vi "Set Ao.vi"(8 "error in (no error)":errorcluster, 9 "Indx":i32, 10 "Value":dbl, 11 "FPGA_Concrete in":refnum<class "FPGA_Concrete.lvclass">) -> (0 "error out":errorcluster, 3 "FPGA_Concrete out":refnum<class "FPGA_Concrete.lvclass">)   [LabVIEW 2019, in "FPGA_Concrete.lvclass"]
uses:
  FPGA_Concrete.lvclass
  FPGA_Concrete.lvclass/FPGA_Concrete.ctl
  <vilib>/Utility/error.llb/Error Cluster From Error Code.vi
  <vilib>/rvi/errors/niLvFpgaAdjustHostInterfaceError.vi
  <vilib>/ErrorRing/Error Ring.xnode
  <vilib>/rvi/interface/nirviReadWriteControl/nirviReadWriteControl.xnode
  FPGA VI Reference.ctl
  NiFpgaLv.dll
  <vilib>/rvi/interface/Simulation/niFpgaSimulationCallBeginRW.vi
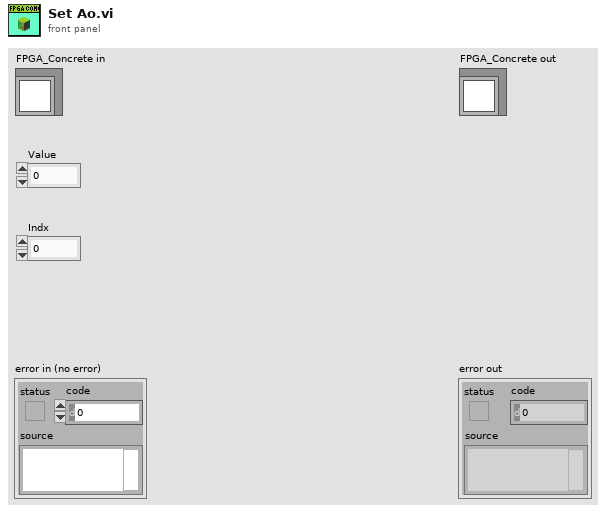
[diagram p1: front panel]
types:
  T1 = typedef "FPGA_Concrete.lvclass/FPGA VI Reference.ctl" = refnum<k20>
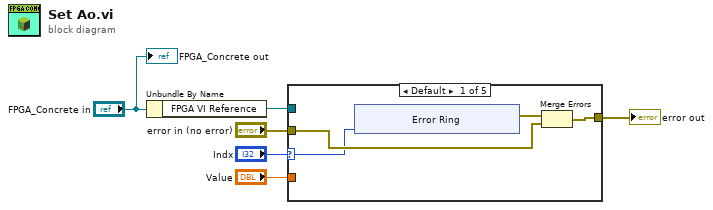
[diagram p0: block diagram]
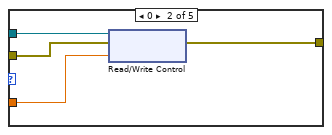
[diagram p2: hidden frame]
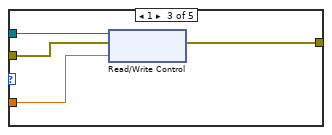
[diagram p3: hidden frame]
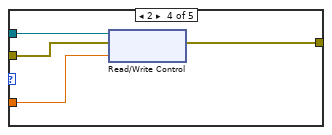
[diagram p4: hidden frame]
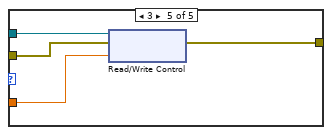
[diagram p5: hidden frame]
diagram:
  n1 = Unbundle By Name("FPGA_Concrete in") -> ("FPGA VI Reference"=w6:T1)
  n2 = case shown="Default" "Indx" {
    selector: "Indx" -> [w9 _ _ _ _]
    tunnel: w6 -> [_ w21 w25 w29 w33]
    tunnel: "error in (no error)" -> [w10 w20 w24 w28 w32]
    tunnel: [w8 w19 w23 w27 w31] -> w3
    tunnel: "Value" -> [_ w18 w22 w26 w30]
    frame Default {
      n3 = xnode "Error Ring"("parameter 0"=w9) -> ("error out"=w7:errorcluster)
      n4 = Merge Errors(w7, w10) -> (w8:errorcluster)
    }
    frame 0 {
      n5 = xnode "Read/Write Control"("FPGA VI Reference In"=w21, "error in"=w20, "Mod5/AO0"=w18) -> ("error out"=w19:errorcluster)  [unwired: 1 out]
    }
    frame 1 {
      n6 = xnode "Read/Write Control"("FPGA VI Reference In"=w25, "error in"=w24, "Mod5/AO1"=w22) -> ("error out"=w23:errorcluster)  [unwired: 1 out]
    }
    frame 2 {
      n7 = xnode "Read/Write Control"("FPGA VI Reference In"=w29, "error in"=w28, "Mod5/AO2"=w26) -> ("error out"=w27:errorcluster)  [unwired: 1 out]
    }
    frame 3 {
      n8 = xnode "Read/Write Control"("FPGA VI Reference In"=w33, "error in"=w32, "Mod5/AO3"=w30) -> ("error out"=w31:errorcluster)  [unwired: 1 out]
    }
  }
  "error out" <- w3
  "FPGA_Concrete out" <- "FPGA_Concrete in"
